vi "Create solenoid.vi"(7 "Variant":variant, 8 "error in (no error)":errorcluster, 9 "Reverse solenoid channel":string, 10 "Forward solenoid channel":string, 11 "Solenoids in":refnum<class "Solenoids.lvclass">) -> (0 "error out":errorcluster, 3 "Solenoids out":refnum<class "Solenoids.lvclass">)   [LabVIEW 2019, in "Pneumatics control.lvlib" / "Pneumatics.lvclass"]
doc: "This VI reads the string keys of the solenoid and sets them to the object using its Begin.vi"
uses:
  Pneumatics.lvclass
  Solenoids/Solenoids.lvclass
  ef8d8219-5e77-4bf2-9fad-3ddeeb6a208f.vi
  012dc745-470c-4ba3-b2ed-ce411de25b11.vi
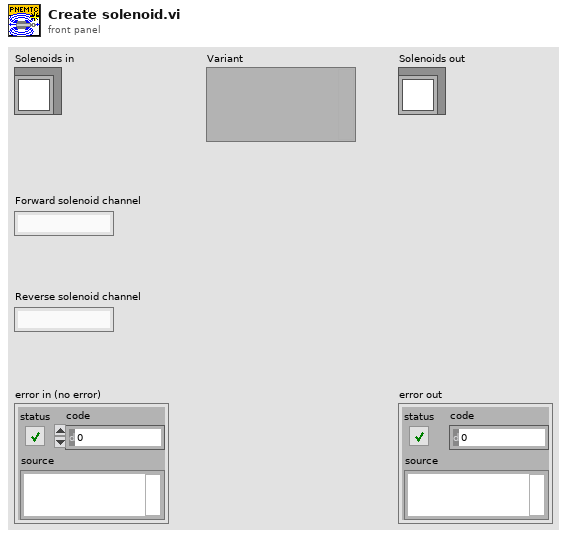
[diagram p1: front panel]
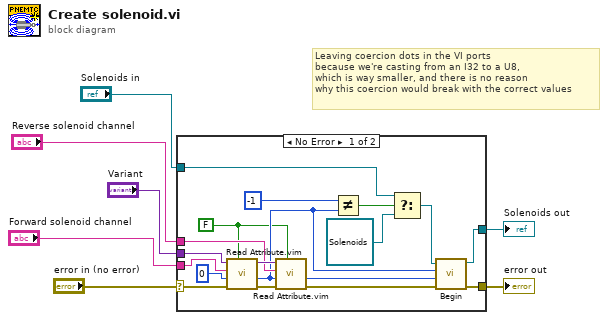
[diagram p0: block diagram]
diagram:
  # "Leaving coercion dots in the VI ports\nbecause we're casting from an I32 to a U8,\nwhich is way smaller, and there is no reason\nwhy this coercion would break with the correct values"
  n1 = case shown="No Error" "error in (no error)" {
    selector: "error in (no error)" -> [w18 w27]
    tunnel: [w25 w27] -> w7
    tunnel: "Variant" -> [w22 _]
    tunnel: "Solenoids in" -> [w11 w26]
    tunnel: [w17 w26] -> w3
    tunnel: "Forward solenoid channel" -> [w16 _]
    tunnel: "Reverse solenoid channel" -> [w15 _]
    frame No Error {
      w8 = FALSE ("Error if not found (T)")
      n2 = call "Read Attribute.vim"("Error if not found (T)"=w8, "error in"=w18, "default value (data type)"=0, "name"=w16, "variant in"=w22) -> ("error out"=w19:errorcluster, "value"=w14:i32, "variant out"=w21:variant)  [unwired: 3 in, 1 out]
      n3 = call "Read Attribute.vim"("Error if not found (T)"=w8, "error in"=w19, "default value (data type)"=w14, "name"=w15, "variant in"=w21) -> ("error out"=w20:errorcluster, "value"=w24:i32)  [unwired: 3 in, 2 out]
      n4 = Not Equal?(x=-1, y=w14) -> (x != y?=w12:bool)
      n5 = Select(t=w11, s=w12, f=refnum<class "Solenoids.lvclass"> refnum) -> (s? t:f=w10:refnum<class "Solenoids.lvclass">)
      n6 = call-dynamic "Begin.vi"("error in (no error)"=w20, "Reverse solenoid channel"=w24, "Forward Solenoid Channel"=w14, "Solenoids in"=w10) -> ("error out"=w25:errorcluster, "Solenoids out"=w17:refnum<class "Solenoids.lvclass">)  [unwired: 6 in]
    }
    frame Error {
    }
  }
  "error out" <- w7
  "Solenoids out" <- w3
